vi "StopLooking.vi"(8 "error in":errorcluster, 10 "stop notif name":string, 11 "SubPanel in":refnum<vi>) -> (0 "error out":errorcluster, 2 "StopAck":bool, 3 "SubPanel out":refnum<vi>)   [LabVIEW 2013, in "FindName Task_Manager.lvlib"]
uses:
  FindName Task_Manager.lvlib
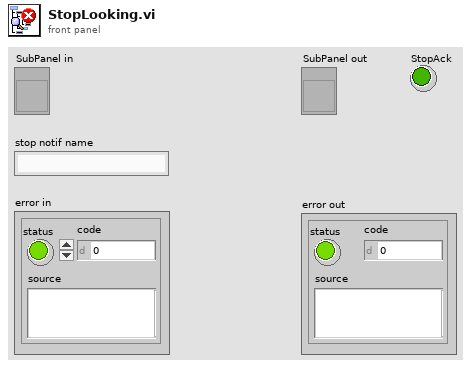
[diagram p1: front panel]
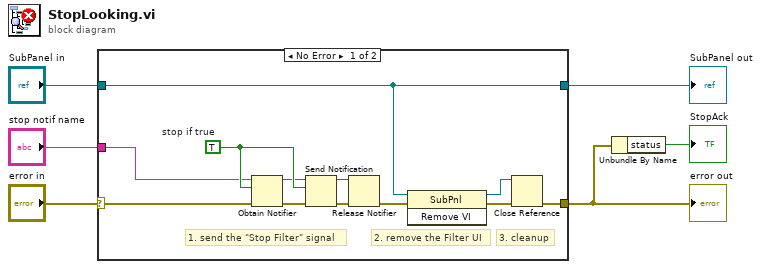
[diagram p0: block diagram]
diagram:
  n1 = case shown="No Error" "error in" {
    selector: "error in" -> [w13 w20]
    tunnel: [w12 w20] -> w5
    tunnel: "SubPanel in" -> [w8 w19]
    tunnel: [w8 w19] -> w2
    tunnel: "stop notif name" -> [w7 _]
    frame No Error {
      w17 = TRUE  # stop if true
      # "3. cleanup"
      # "2. remove the Filter UI"
      # "1. send the \"Stop Filter\" signal"
      n2 = Obtain Notifier(name (unnamed)=w7, notification data type=w17, error in (no error)=w13) -> (notifier out=w14:refnum<notifier>, error out=w15:errorcluster)  [unwired: 1 in, 1 out]
      n3 = Send Notification(notification=w17, notifier=w14, error in (no error)=w15) -> (notifier out=w9:refnum<notifier>, error out=w16:errorcluster)
      n4 = Release Notifier(notifier=w9, error in (no error)=w16) -> (error out=w10:errorcluster)  [unwired: 1 in, 2 out]
      n5 = invoke on="Invoke Node" class="SubPnl" method="Remove VI"(reference=w8, error in=w10) -> (reference out=w11:refnum<vi>, error out=w18:errorcluster)  [unwired: 1 in, 1 out]
      n6 = Close Reference(reference=w11, error in (no error)=w18) -> (error out=w12:errorcluster)
    }
    frame Error {
    }
  }
  "error out" <- w5
  "SubPanel out" <- w2
  n7 = Unbundle By Name(w5) -> ("status"=→"StopAck":bool)
